vi "testCalcEffGQFWHM.vi"(8 "error in (no error)":errorcluster) -> (0 "error out":errorcluster)   [LabVIEW 2016]
doc: "Test to calculate the effective FWHM by Gaussian quadrature."
uses:
  OptCtrl/OptCtrl.lvclass
  StrictDef/InstName.ctl
  MatOper/getSubArray2D.vi
  OfcFunc.lvlib
  MatOper/MatOper.lvclass
  <vilib>/addons/_JKI Toolkits/Caraya/classes/Test/Test.lvclass
  <vilib>/addons/_JKI Toolkits/Caraya/classes/Assert/Assert.lvclass
panel:
  in  "OfcFunc.lvlib:OptCtrl.lvclass":refnum<class "OptCtrl.lvclass">
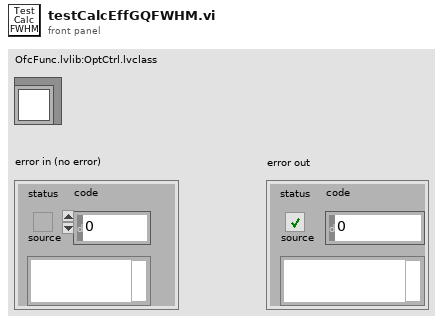
[diagram p1: front panel]
types:
  T1 = typedef "OfcFunc.lvlib/InstName.ctl" = enum16{"lsst", "comcam"}
  T2 = cluster{"Config Dir":path, "Config File Name":string, "Inst Name":T1, "State 0 File Name":string, "Weighting File Name":string, "PSSN Alpha File Name":string, "Authority Files":cluster{"Rigid Body Stroke File":string, "M1M3 Subsystem":cluster{"Mirror":string, "Actuatro Force File":string}, "M2 Subsystem":cluster{"Mirror":string, "Actuatro Force File":string}, "Num of Bending Mode":i32}}
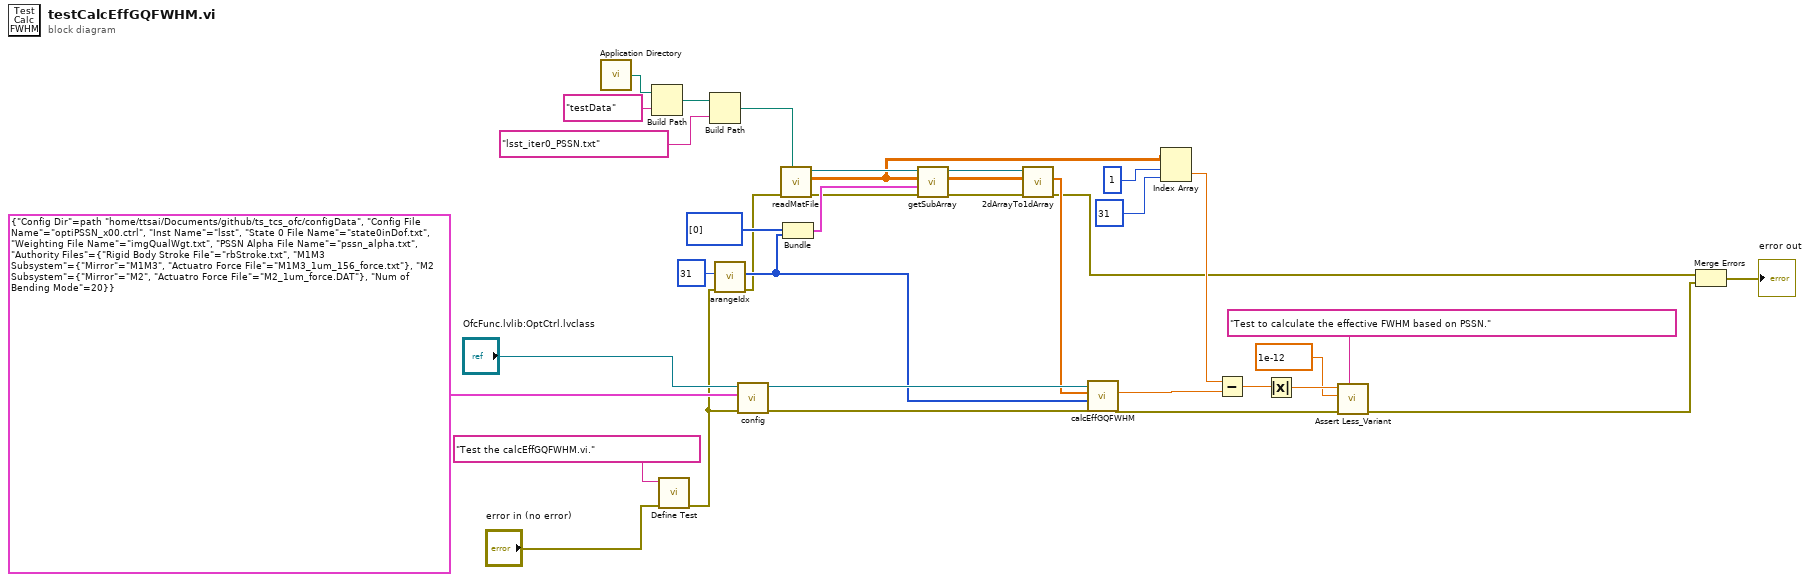
[diagram p0: block diagram]
diagram:
  n1 = call <vilib>:"Application Directory.vi"() -> ("Application Directory"=w34:path)
  n2 = Build Path(base path=w34, name or relative path="testData") -> (appended path=w32:path)
  n3 = call <vilib>:"Define Test.vi"("error in (no error)"="error in (no error)", "Label (VI Title)"="Test the calcEffGQFWHM.vi.") -> ("error out"=w8:errorcluster)  [unwired: 9 in]
  n4 = Build Path(base path=w32, name or relative path="lsst_iter0_PSSN.txt") -> (appended path=w30:path)
  n5 = call "arangeIdx.vi"("error in (no error)"=w8, "Number"=31) -> ("error out"=w12:errorcluster, "Idx Array"=w21:i32[])  [unwired: 7 in, 1 out]
  n6 = call "config.vi"("error in (no error)"=w8, "Configuration"=T2 {"Config Dir"=path "/home/ttsai/Documents/github/ts_tcs_ofc/configData", "Config File Name"="optiPSSN_x00.ctrl", "Inst Name"=enum."lsst", "State 0 File Name"="state0inDof.txt", "Weighting File Name"="imgQualWgt.txt", "PSSN Alpha File Name"="pssn_alpha.txt", "Authority Files"={"Rigid Body Stroke File"="rbStroke.txt", "M1M3 Subsystem"={"Mirror"="M1M3", "Actuatro Force File"="M1M3_1um_156_force.txt"}, "M2 Subsystem"={"Mirror"="M2", "Actuatro Force File"="M2_1um_force.DAT"}, "Num of Bending Mode"=20}}, "OptCtrl in"="OfcFunc.lvlib:OptCtrl.lvclass") -> ("error out"=w9:errorcluster, "OptCtrl out"=w25:refnum<class "OptCtrl.lvclass">)  [unwired: 7 in]
  n7 = call "readMatFile.vi"("Path"=w30, "error in (no error)"=w12) -> ("error out"=w11:errorcluster, "Matrix"=w20:dbl[][], "MatOper out"=w29:refnum<class "MatOper.lvclass">)  [unwired: 7 in]
  n8 = Bundle(i32[] [0], "Idx Array"=w21) -> (w26:cluster{i32[], "Idx Array":i32[]})  [unwired: 1 in]
  n9 = call-poly "getSubArray.vi"("error in (no error)"=w11, "Index Array Cluster"=w26, "2D Array"=w20, "MatOper in"=w29) -> ("error out"=w10:errorcluster, "Sub-Array"=w24:dbl[][], "MatOper out"=w22:refnum<class "MatOper.lvclass">)  [unwired: 5 in]
  n10 = call "2dArrayTo1dArray.vi"("error in (no error)"=w10, "2D Array"=w24, "MatOper in"=w22) -> ("error out"=w4:errorcluster, "1D Array"=w23:dbl[])  [unwired: 6 in, 1 out]
  n11 = call "calcEffGQFWHM.vi"("error in (no error)"=w9, "Field Idx"=w21, "PSSN"=w23, "OptCtrl in"=w25) -> ("error out"=w5:errorcluster, "Effective GQFWHM (arcsec)"=w16:dbl)  [unwired: 5 in, 1 out]
  n12 = Index Array(array=w20, index (row)=1, index (col)=31 ("disabled index (col)")) -> (element=w17:dbl)
  n13 = Subtract(x=w17, y=w16) -> (x-y=w15:dbl)
  n14 = Absolute Value(x=w15) -> (abs(x)=w7:dbl)
  n15 = call <vilib>:"Assert Less_Variant.vi"("Label"="Test to calculate the effective FWHM based on PSSN.", "error in (no error)"=w5, "Y"=1e-12, "X"=w7) -> ("error out"=w3:errorcluster)  [unwired: 7 in]
  n16 = Merge Errors(w4, w3) -> (→"error out":errorcluster)
